vi "Writing X Galvo Voltages.vi"() -> ()   [LabVIEW 2018]
uses:
  <resource>/objmgr/daqmx.rc
  <vilib>/DAQmx/create/channels.llb/DAQmx Create Channel (AO-Voltage-Basic).vi
  <vilib>/DAQmx/configure/timing.llb/DAQmx Timing (Sample Clock).vi
  <vilib>/DAQmx/write.llb/DAQmx Write (Analog 1D DBL 1Chan NSamp).vi
  <vilib>/DAQmx/write.llb/DAQmx Write (Counter Ticks 1Chan 1Samp).vi
  <vilib>/DAQmx/create/channels.llb/DAQmx Create Channel (CO-Pulse Generation-Ticks).vi
  <vilib>/DAQmx/configure/events/hardwareSignals.llb/DAQmx Export Signal (Most Signals).vi
  <vilib>/DAQmx/create/channels.llb/DAQmx Create Channel (CI-Count Edges).vi
panel:
  out "error out":errorcluster
  in  "data":dbl[](array[numeric]) format="%0.2f"
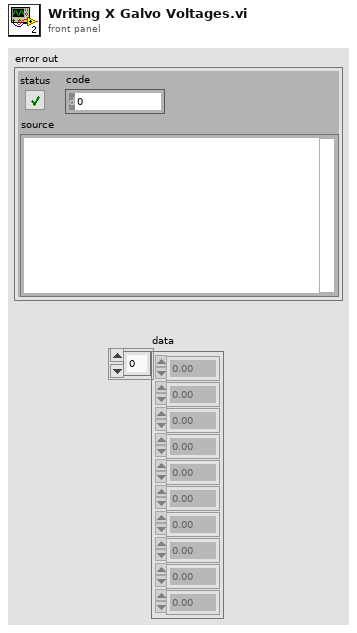
[diagram p1: front panel]
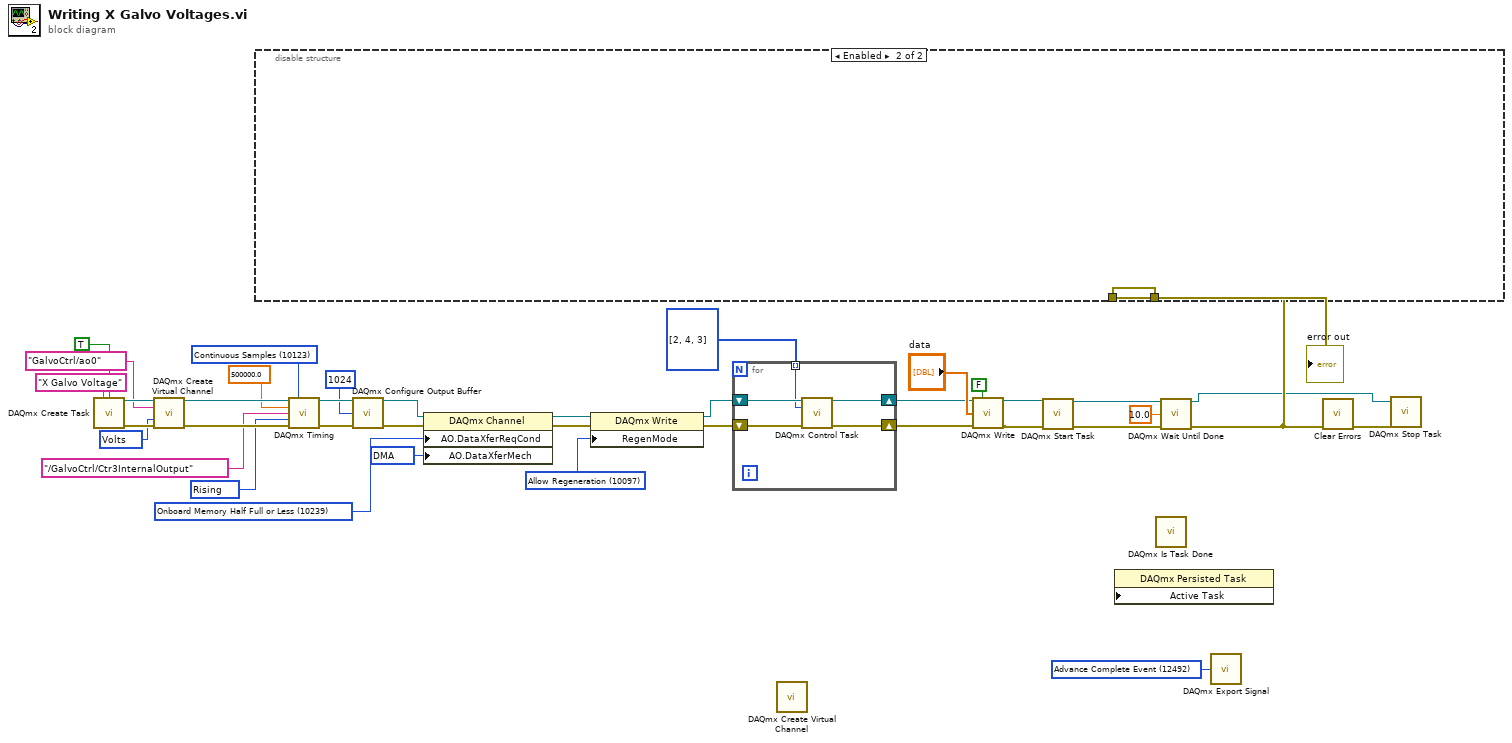
[diagram p0: block diagram]
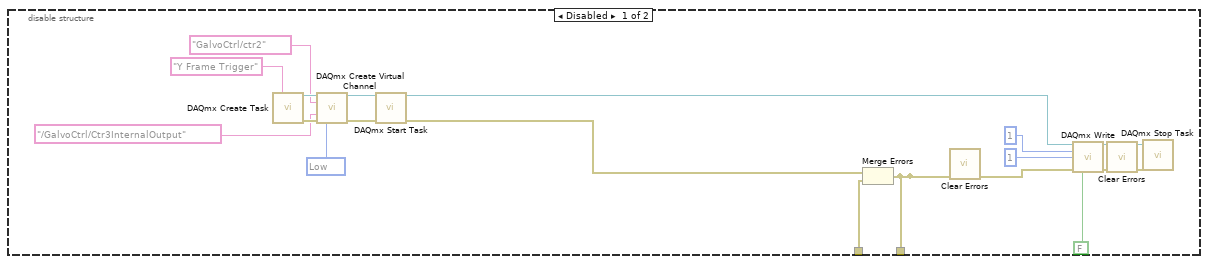
[diagram p2: hidden frame]
diagram:
  w1 = 12492 items=["AI Convert Clock"=12484, "10MHz Reference Clock"=12536, "20MHz Timebase Clock"=12486, "Sample Clock"=12487, "Advance Trigger"=12488, "Reference Trigger"=12490, "Start Trigger"=12491, "Advance Complete Event"=12492, "AI Hold Complete Event"=12493, "Counter Output Event"=12494, "Change Detection Event"=12511, "Watchdog Timer Expired Event"=12512] ("signal")
  w12 = 10054 items=["DMA"=10054, "Interrupts"=10204, "Programmed I/O"=10264, "USB Bulk"=12590] ("AO.DataXferMech")
  w13 = 10239 items=["Onboard Memory Empty"=10235, "Onboard Memory Half Full or Less"=10239, "Onboard Memory Less than Full"=10242] ("AO.DataXferReqCond")
  w21 = 10123 items=["Finite Samples"=10178, "Continuous Samples"=10123, "Hardware Timed Single Point"=12522] ("sample mode")
  w27 = 10280 items=["Rising"=10280, "Falling"=10171] ("active edge")
  w32 = i32[] [2, 4, 3] items=["verify"=2, "reserve"=4, "commit"=3, "unreserve"=5, "abort"=6]
  w33 = 10097 items=["Allow Regeneration"=10097, "Do Not Allow Regeneration"=10158] ("RegenMode")
  w35 = 10348 items=["Volts"=10348, "From Custom Scale"=10065] ("units")
  n1 = call <vilib>:"DAQmx Create Task.vi"("new task name"="X Galvo Voltage", "auto cleanup"=TRUE) -> ("task out"=w38:refnum<k21>, "error out"=w37:errorcluster)  [unwired: 12 in]
  n2 = call-poly <vilib>:"DAQmx Create Virtual Channel.vi"("task in"=w38, "physical channels"=tag "GalvoCtrl/ao0", "units"=w35, "error in"=w37) -> ("task out"=w31:refnum<k21>, "error out"=w34:errorcluster)  [unwired: 10 in]
  n3 = call-poly <vilib>:"DAQmx Timing.vi"("task/channels in"=w31, "sample mode"=w21, "rate"=500000.0, "source"=tag "/GalvoCtrl/Ctr3InternalOutput" ("source of ticks"), "active edge"=w27, "error in"=w34) -> ("task out"=w16:refnum<k21>, "error out"=w28:errorcluster)  [unwired: 8 in]
  n4 = call <vilib>:"DAQmx Configure Output Buffer.vi"("task/channels in"=w16, "buffer size (in samples per channel)"=u32 1024, "error in"=w28) -> ("task out"=w10:refnum<k21>, "error out"=w17:errorcluster)  [unwired: 11 in]
  n5 = property class="DAQmx Channel"(reference=w10, error in=w17, "AO.DataXferReqCond"=w13, "AO.DataXferMech"=w12) -> (reference out=w11:refnum<k21>, error out=w14:errorcluster)
  n6 = property class="DAQmx Write"(reference=w11, error in=w14, "RegenMode"=w33) -> (reference out=w25:refnum<k21>, error out=w26:errorcluster)
  n7 = for {
    shift-right: [w43] -> w9
    shift-left: w26 -> [w44]
    tunnel: w32 -> [w41] mode=indexing
    shift-right: [w40] -> w8
    shift-left: w25 -> [w42]
    n8 = call <vilib>:"DAQmx Control Task.vi"("task/channels in"=w42, "action"=w41, "error in"=w44) -> ("task out"=w40:refnum<k21>, "error out"=w43:errorcluster)  [unwired: 11 in]
  }
  n9 = call-poly <vilib>:"DAQmx Create Virtual Channel.vi"() -> ()  [unwired: 14 in, 2 out]
  n10 = call-poly <vilib>:"DAQmx Write.vi"("task/channels in"=w8, "auto start"=FALSE, "data"="data", "error in"=w9) -> ("task out"=w6:refnum<k21>, "error out"=w22:errorcluster)  [unwired: 9 in, 1 out]
  n11 = call <vilib>:"DAQmx Start Task.vi"("task/channels in"=w6, "error in"=w22) -> ("task out"=w4:refnum<k21>, "error out"=w7:errorcluster)  [unwired: 12 in]
  n12 = property class="DAQmx Persisted Task" props=["Active Task"]() -> ()  [unwired: 3 in, 2 out]
  n13 = call <vilib>:"DAQmx Is Task Done.vi"() -> ()  [unwired: 13 in, 3 out]
  n14 = call <vilib>:"DAQmx Wait Until Done.vi"("task/channels in"=w4, "timeout (sec)"=10.0, "error in"=w7) -> ("task out"=w2:refnum<k21>, "error out"=w5:errorcluster)  [unwired: 11 in]
  n15 = disable-structure shown="Enabled" {
    disable-tunnel: w5 -> [w49 w64]
    disable-tunnel: [w45 w64] -> w19
    frame Disabled {
      w55 = 10214 items=["High"=10192, "Low"=10214] ("idle state")
      n16 = call <vilib>:"DAQmx Create Task.vi"("new task name"="Y Frame Trigger") -> ("task out"=w57:refnum<k21>, "error out"=w58:errorcluster)  [unwired: 13 in]
      n17 = call-poly <vilib>:"DAQmx Create Virtual Channel.vi"("task in"=w57, "counter"=tag "GalvoCtrl/ctr2", "source of ticks"=tag "/GalvoCtrl/Ctr3InternalOutput", "error in"=w58, "idle state"=w55) -> ("task out"=w54:refnum<k21>, "error out"=w53:errorcluster)  [unwired: 9 in]
      n18 = call <vilib>:"DAQmx Start Task.vi"("task/channels in"=w54, "error in"=w53) -> ("task out"=w61:refnum<k21>, "error out"=w50:errorcluster)  [unwired: 12 in]
      n19 = Merge Errors(w50, w49) -> (w45:errorcluster)
      n20 = call <vilib>:"Clear Errors.vi"("error in (no error)"=w45) -> ("error out"=w47:errorcluster)  [unwired: 5 in, 1 out]
      n21 = call-poly <vilib>:"DAQmx Write.vi"("task/channels in"=w61, "auto start"=FALSE, "high ticks"=u32 1, "low ticks"=u32 1, "error in"=w47) -> ("task out"=w51:refnum<k21>, "error out"=w52:errorcluster)  [unwired: 8 in, 1 out]
      n22 = call <vilib>:"Clear Errors.vi"("error in (no error)"=w52) -> ("error out"=w46:errorcluster)  [unwired: 5 in, 1 out]
      n23 = call <vilib>:"DAQmx Stop Task.vi"("task/channels in"=w51, "error in"=w46) -> ()  [unwired: 12 in, 2 out]
    }
    frame Enabled {
    }
  }
  "error out" <- w19
  n24 = call-poly <vilib>:"DAQmx Export Signal.vi"("signal"=w1) -> ()  [unwired: 13 in, 2 out]
  n25 = call <vilib>:"Clear Errors.vi"("error in (no error)"=w5) -> ("error out"=w20:errorcluster)  [unwired: 5 in, 1 out]
  n26 = call <vilib>:"DAQmx Stop Task.vi"("task/channels in"=w2, "error in"=w20) -> ()  [unwired: 12 in, 2 out]
